vi "Read U64.vi"(8 "error in":errorcluster, 9 "RegisterOffset":u32, 10 "register name":string, 11 "session in":u32) -> (0 "error out":errorcluster, 2 "value out":u64, 3 "session out":u32)   [LabVIEW 2024, in "FPGA Register IO.lvlib"]
uses:
  FPGA Register IO.lvlib
  NiFpga.dll
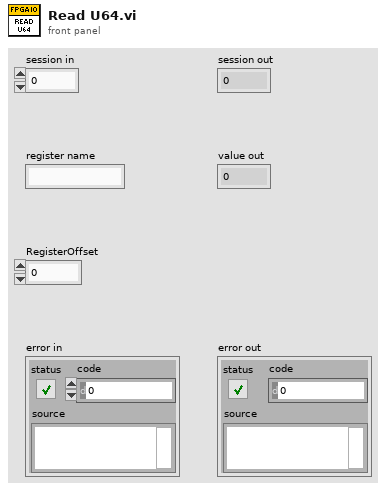
[diagram p1: front panel]
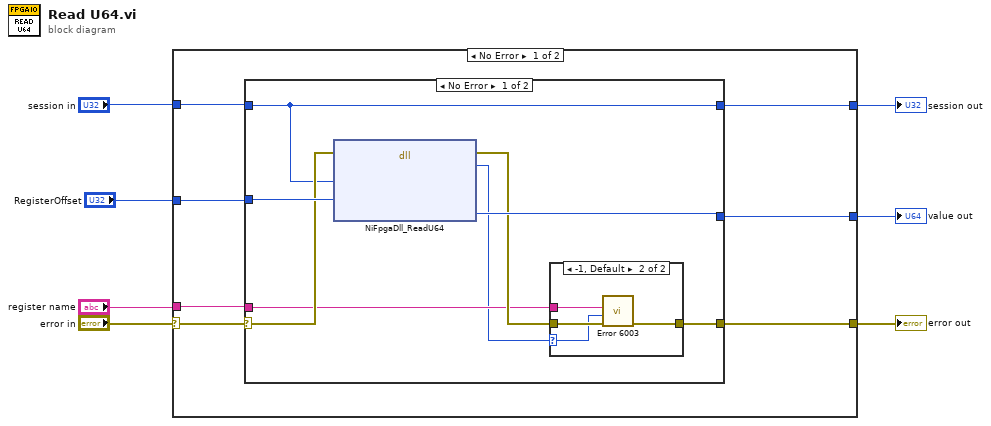
[diagram p0: block diagram]
diagram:
  n1 = case shown="No Error" "error in" {
    selector: "error in" -> [w8 w31]
    tunnel: [w14 w31] -> w7
    tunnel: [w13 _] -> w6
    tunnel: [w12 w30] -> w5
    tunnel: "session in" -> [w9 w30]
    tunnel: "register name" -> [w11 _]
    tunnel: "RegisterOffset" -> [w10 _]
    frame No Error {
      n2 = case shown="No Error" w8 {
        selector: w8 -> [w20 w29]
        tunnel: w9 -> [w19 w28]
        tunnel: [w18 w29] -> w14
        tunnel: [w22 _] -> w13
        tunnel: w10 -> [w21 _]
        tunnel: [w19 w28] -> w12
        tunnel: w11 -> [w16 _]
        frame No Error {
          n3 = dll-call lib="NiFpga.*" fn="NiFpgaDll_ReadU64"(error in=w20, "session"=w19, "offset"=w21) -> (error out=w17:errorcluster, "status"=w15:i32, "value"=w22:u64)  [unwired: 5 in, 1 out]
          n4 = case shown="-1, Default" w15 {
            selector: w15 -> [_ w24]
            tunnel: w17 -> [w23 w27]
            tunnel: [w23 w26] -> w18
            tunnel: w16 -> [_ w25]
            frame 0 {
            }
            frame -1, Default {
              n5 = call "Error 6003.vi"("error in (no error)"=w27, "rio status code"=w24, "register name"=w25) -> ("error out"=w26:errorcluster)  [unwired: 8 in]
            }
          }
        }
        frame Error {
        }
      }
    }
    frame Error {
    }
  }
  "error out" <- w7
  "session out" <- w5
  "value out" <- w6
